vi "filterWheelGetPosition.vi"() -> (0 "number":i32)   [LabVIEW 2017]
uses:
  globalDevices.vi
panel:
  out "substring":string
  out "read buffer":string
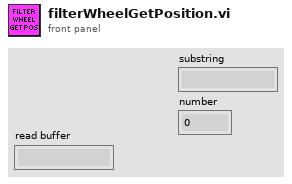
[diagram p1: front panel]
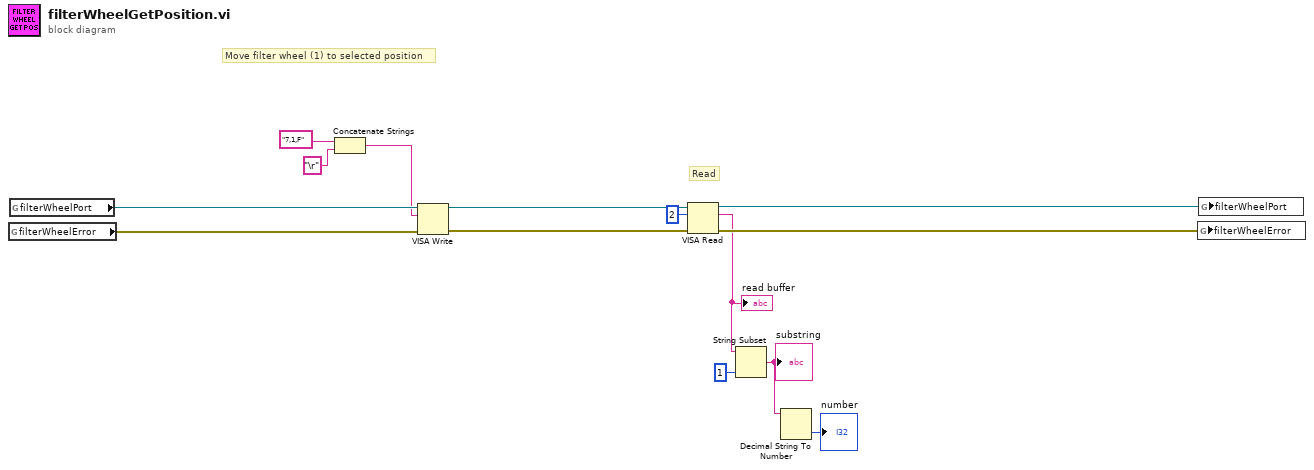
[diagram p0: block diagram]
diagram:
  # "Read"
  # "Move filter wheel (1) to selected position"
  n1 = global read "globalDevices.vi" "filterWheelError"() -> (w13:errorcluster)
  n2 = global read "globalDevices.vi" "filterWheelPort"() -> (w14:refnum<visa-resource-name>)
  n3 = Concatenate Strings("7,1,F", "\r" ("string")) -> (w11:string)
  n4 = VISA Write(VISA resource name=w14, write buffer=w11, error in (no error)=w13) -> (VISA resource name out=w10:refnum<visa-resource-name>, error out=w9:errorcluster)  [unwired: 1 out]
  n5 = VISA Read(VISA resource name=w10, byte count=u32 2, error in (no error)=w9) -> (VISA resource name out=w8:refnum<visa-resource-name>, read buffer=w4:string, error out=w7:errorcluster)  [unwired: 1 out]
  "read buffer" <- w4
  n6 = String Subset(string=w4, length (rest)=1 ("length (rest)")) -> (substring=w2:string)  [unwired: 1 in]
  "substring" <- w2
  n7 = Decimal String To Number(string=w2) -> (number=→"number":i32)  [unwired: 2 in, 1 out]
  n8 = global write "globalDevices.vi" "filterWheelError"(w7) -> ()
  n9 = global write "globalDevices.vi" "filterWheelPort"(w8) -> ()
